vi "Read ChannelName.vi"(8 "error in (no error)":errorcluster, 11 "9770 API in":refnum<class "9770 API.lvclass">) -> (0 "error out":errorcluster, 2 "ChannelName":string, 3 "9770 API out":refnum<class "9770 API.lvclass">)   [LabVIEW 2017, in "9770 API.lvclass"]
uses:
  <vilib>/addons/InsightCM/Devices/Shared/Emsa/Emsa9770API/9770 API.lvclass
  <vilib>/addons/InsightCM/Devices/Shared/Emsa/Emsa9770API/9770 API.lvclass/9770 API.ctl
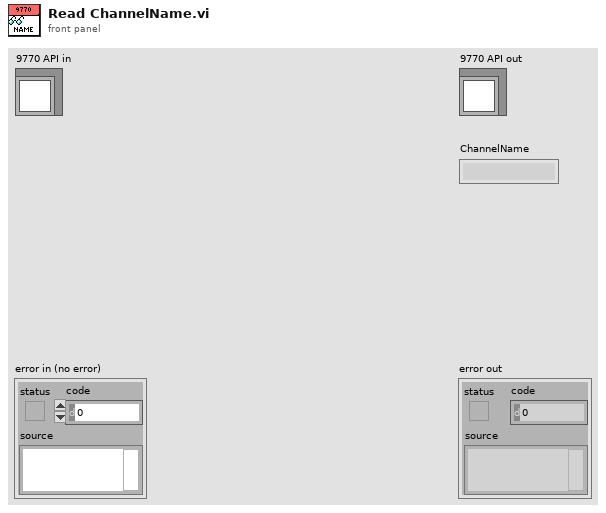
[diagram p1: front panel]
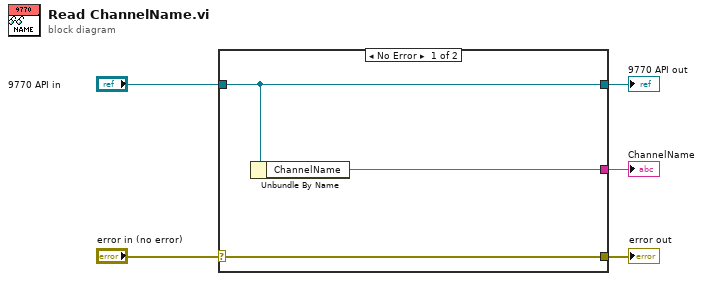
[diagram p0: block diagram]
diagram:
  n1 = case shown="No Error" "error in (no error)" {
    selector: "error in (no error)" -> [w8 w9]
    tunnel: [w8 w9] -> w4
    tunnel: [w7 w10] -> w2
    tunnel: "9770 API in" -> [w7 w10]
    tunnel: [w6 _] -> w1
    frame No Error {
      n2 = Unbundle By Name(w7) -> ("ChannelName"=w6:string)
    }
    frame Error {
    }
  }
  "error out" <- w4
  "9770 API out" <- w2
  "ChannelName" <- w1
